vi "Load Glyph from File.vi"(8 "error in (no error)":errorcluster) -> (0 "error out":errorcluster, 1 "file name":string, 2 "Pic Out":picture, 4 "Canceled?":bool)   [LabVIEW 2021]
uses:
  <vilib>/LabVIEW Icon API/lv_icon/lv_icon.lvlib
panel:
  in  "ErrorMessage":string="%s is not a supported file type.  Please use a BMP, JPG, or PNG file."
  in  "Localized 2":string="Choose a graphic to import"
  in  "Localized":string="Glyph"
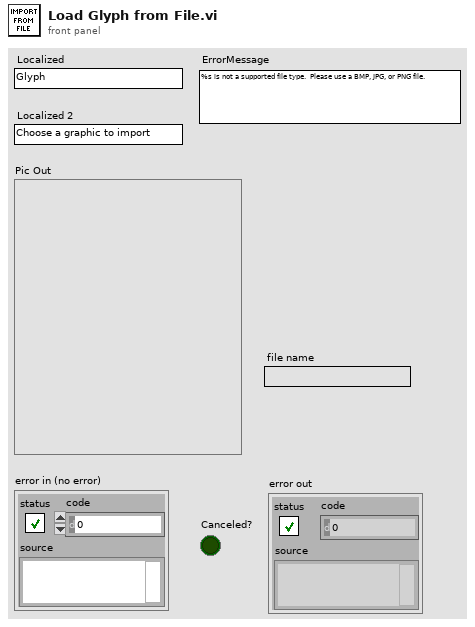
[diagram p1: front panel]
types:
  T1 = typedef "imagedata.ctl" = cluster{"image type":i32, "image depth":i32, "image":u8[], "mask":u8[], "colors":u32[], "Rectangle":cluster{"left":i16, "top":i16, "right":i16, "bottom":i16}}
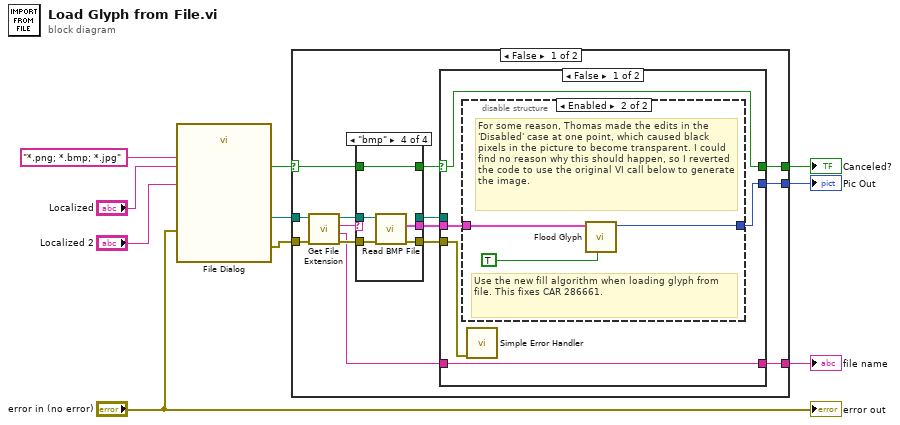
[diagram p0: block diagram]
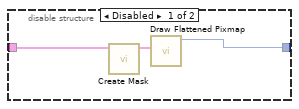
[diagram p2: hidden frame]
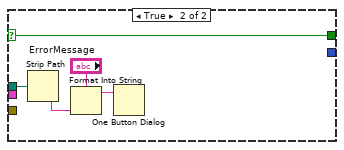
[diagram p3: hidden frame]
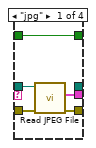
[diagram p4: hidden frame]
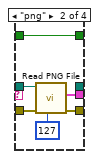
[diagram p5: hidden frame]
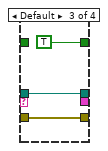
[diagram p6: hidden frame]
diagram:
  n1 = call "File Dialog"("prompt"="Localized 2", "error in"="error in (no error)", "pattern (all files)"="*.png; *.bmp; *.jpg", "pattern label"="Localized") -> ("selected path"=w7:path, "cancelled"=w5:bool, "error out"=w6:errorcluster)  [unwired: 8 in, 1 out]
  n2 = case shown="False" w5 {
    selector: w5 -> [w16 w60]
    tunnel: w7 -> [w24 _]
    tunnel: w6 -> [w23 _]
    tunnel: [w17 _] -> w4
    tunnel: [w12 _] -> w3
    tunnel: [w14 w60] -> w2
    frame False {
      n3 = call <vilib>:"Get File Extension.vi"("error in (no error)"=w23, "file"=w24) -> ("error out"=w22:errorcluster, "filename without extension"=w13:string, "lowercase file extension"=w20:string, "dup file"=w21:path)  [unwired: 5 in, 1 out]
      n4 = case shown="\"bmp\"" w20 {
        tunnel: w22 -> [w45 w50 w54 w59]
        tunnel: [w44 w51 w54 w58] -> w19
        tunnel: [w43 w49 _ w57] -> w18
        tunnel: w21 -> [w42 w48 w52 w56]
        tunnel: w16 -> [w41 w46 _ w55]
        tunnel: [w41 w46 TRUE w55] -> w15
        tunnel: [_ _ w52 _] -> w11
        frame "jpg" {
          n5 = call <vilib>:"Read JPEG File.vi"("error in (no error)"=w45, "path to JPEG file"=w42) -> ("error out"=w44:errorcluster, "image data"=w43:T1)  [unwired: 8 out]
        }
        frame "png" {
          n6 = call <vilib>:"Read PNG File.vi"("Transparency Thresh"=u8 127, "error in (no error)"=w50, "path to PNG file"=w48) -> ("error out"=w51:errorcluster, "image data"=w49:T1)  [unwired: 7 out]
        }
        frame Default {
        }
        frame "bmp" {
          n7 = call <vilib>:"Read BMP File.vi"("error in (no error)"=w59, "path to BMP file"=w56) -> ("error out"=w58:errorcluster, "image data"=w57:T1)  [unwired: 8 out]
        }
      }
      n8 = case shown="False" w15 {
        selector: w15 -> [w26 w40]
        tunnel: w19 -> [w29 _]
        tunnel: w18 -> [w28 _]
        tunnel: [w25 _] -> w17
        tunnel: [w26 w40] -> w14
        tunnel: w13 -> [w27 _]
        tunnel: [w27 _] -> w12
        tunnel: w11 -> [_ w39]
        frame False {
          n9 = disable-structure shown="Enabled" {
            disable-tunnel: w28 -> [w31 w35]
            disable-tunnel: [w30 w34] -> w25
            frame Disabled {
              n10 = call <vilib>:"Create Mask.vi"("image data"=w31) -> ("image data"=w32:T1)  [unwired: 3 in, 7 out]
              n11 = call <vilib>:"Draw Flattened Pixmap.vi"("image data"=w32) -> ("new picture"=w30:picture)  [unwired: 1 in, 7 out]
            }
            frame Enabled {
              # "Use the new fill algorithm when loading glyph from file. This fixes CAR 286661."
              # "For some reason, Thomas made the edits in the 'Disabled' case at one point, which caused black pixels in the picture to become transparent. I could find no reason why this should happen, so I reverted the code to use the original VI call below to generate the image."
              n12 = call <vilib>:"Flood Glyph.vi"("Use New Fill Algorithm? (F)"=TRUE, "image data"=w35) -> ("Pic Out"=w34:picture)  [unwired: 9 out]
            }
          }
          n13 = call <vilib>:"Simple Error Handler.vi"("error in (no error)"=w29) -> ()  [unwired: 4 in, 5 out]
        }
        frame True {
          n14 = Strip Path(path=w39) -> (name=w37:string)  [unwired: 1 out]
          n15 = Format Into String(format string="ErrorMessage", w37) -> (resulting string=w36:string)  [unwired: 2 in, 1 out]
          n16 = One Button Dialog(message=w36) -> ()  [unwired: 1 in, 1 out]
        }
      }
    }
    frame True {
    }
  }
  "Canceled?" <- w2
  "Pic Out" <- w4
  "file name" <- w3
  "error out" <- "error in (no error)"
